vi "gfitsio-format-date-time-string.vi"(10 "timestamp":timestamp) -> (2 "date/time string":string)   [LabVIEW 2023, in "gfitsio.lvlib"]
doc: "Formats a LabVIEW timestamp value into a 23 character date-time string using the following format: YYYY-MM-DDTHH:MM:SS.SSS where\n\nYYYY -- Four digit year\nMM -- Two digit month\nDD -- Two digit day of month\nT -- Literal separator\nHH -- Two digit hour using 24-hour format\nMM -- Two digit minute\nSS.SSS -- Two digit seconds to millisecond precision"
uses:
  gfitsio.lvlib
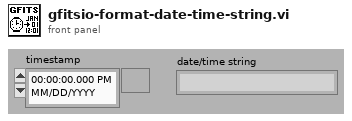
[diagram p1: front panel]
types:
  T1 = cluster{"second":i32, "minute":i32, "hour":i32, "day of month":i32, "month":i32, "year":i32, "day of week":i32, "day of year":i32, "is DST":i32}
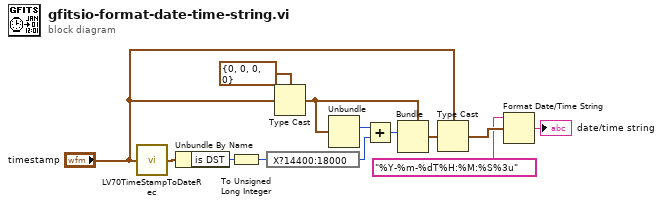
[diagram p0: block diagram]
diagram:
  n1 = call <vilib>:"LV70TimeStampToDateRec.vi"("time stamp"="timestamp") -> ("date time rec"=w3:T1)
  n2 = Unbundle By Name(w3) -> ("is DST"=w4:i32)
  n3 = To Unsigned Long Integer(number=w4) -> (unsigned 32bit integer=w8:u32)
  n4 = expression code="X?14400:18000"(w8) -> (w7:u32)
  n5 = Type Cast(type=cluster{u32, u32, u32, u32} {0, 0, 0, 0}, x="timestamp") -> (*(type *) &x=w9:cluster{u32, u32, u32, u32})
  n6 = Unbundle(w9) -> (w6:u32)  [unwired: 3 out]
  n7 = Add(x=w6, y=w7) -> (x+y=w10:u32)
  n8 = Bundle(cluster=w9, w10) -> (w11:cluster{u32, u32, u32, u32})  [unwired: 3 out]
  n9 = Type Cast(type="timestamp", x=w11) -> (*(type *) &x=w12:timestamp)
  n10 = Format Date/Time String(time format string (%c)="%Y-%m-%dT%H:%M:%S%3u", seconds (now)=w12) -> (date/time string=→"date/time string":string)  [unwired: 1 out]
